vi "Is Closed.vi"(11 "Writer in":refnum<class "Writer.lvclass">) -> (2 "Is Closed?":bool)   [LabVIEW 2022 SP3, in "Enclave.lvlib" / "Writer.lvclass"]
uses:
  Writer.lvclass
  Writer.lvclass/Writer.ctl
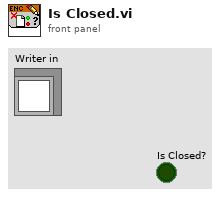
[diagram p1: front panel]
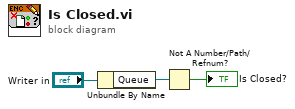
[diagram p0: block diagram]
diagram:
  n1 = Unbundle By Name("Writer in") -> ("Queue"=w2:refnum<queue>)
  n2 = Not A Number/Path/Refnum?(number/path/refnum=w2) -> (NaN/Path/Refnum?=→"Is Closed?":bool)
